vi "prevodni_charakteristika.vi"() -> ()   [LabVIEW 2024]
uses:
  <vilib>/Analysis/baseanly.llb/Mean (DBL).vi
  <instrlib>/EFmeter/EFmeter.lvlib
  <vilib>/Analysis/NI_AALBase.lvlib
panel:
  in  "Dalsi krok\nDalsikrok":bool
  in  "Zpusob rizeni napeti":u16(ring) items=["Sweep", "Manualni", ""]
  in  "VISA EFmeter":refnum<visa-resource-name>
  out "S":dbl
  in  "file path (use dialog)":path
  in  "Prodleva mezi vzorky(ms)":u32
  in  "Prumerovani":bool
  in  "Vzorku na kroků":u16 max=100 step=1
  out "Prevodni charakteristika":cluster{"X":dbl[], "Y":dbl[]}[](graph)
  in  "Clear":bool
  in  "Uložit data":bool
  in  "Start":bool
  in  "VISA  zdroj":refnum<visa-resource-name>
  in  "stop":bool
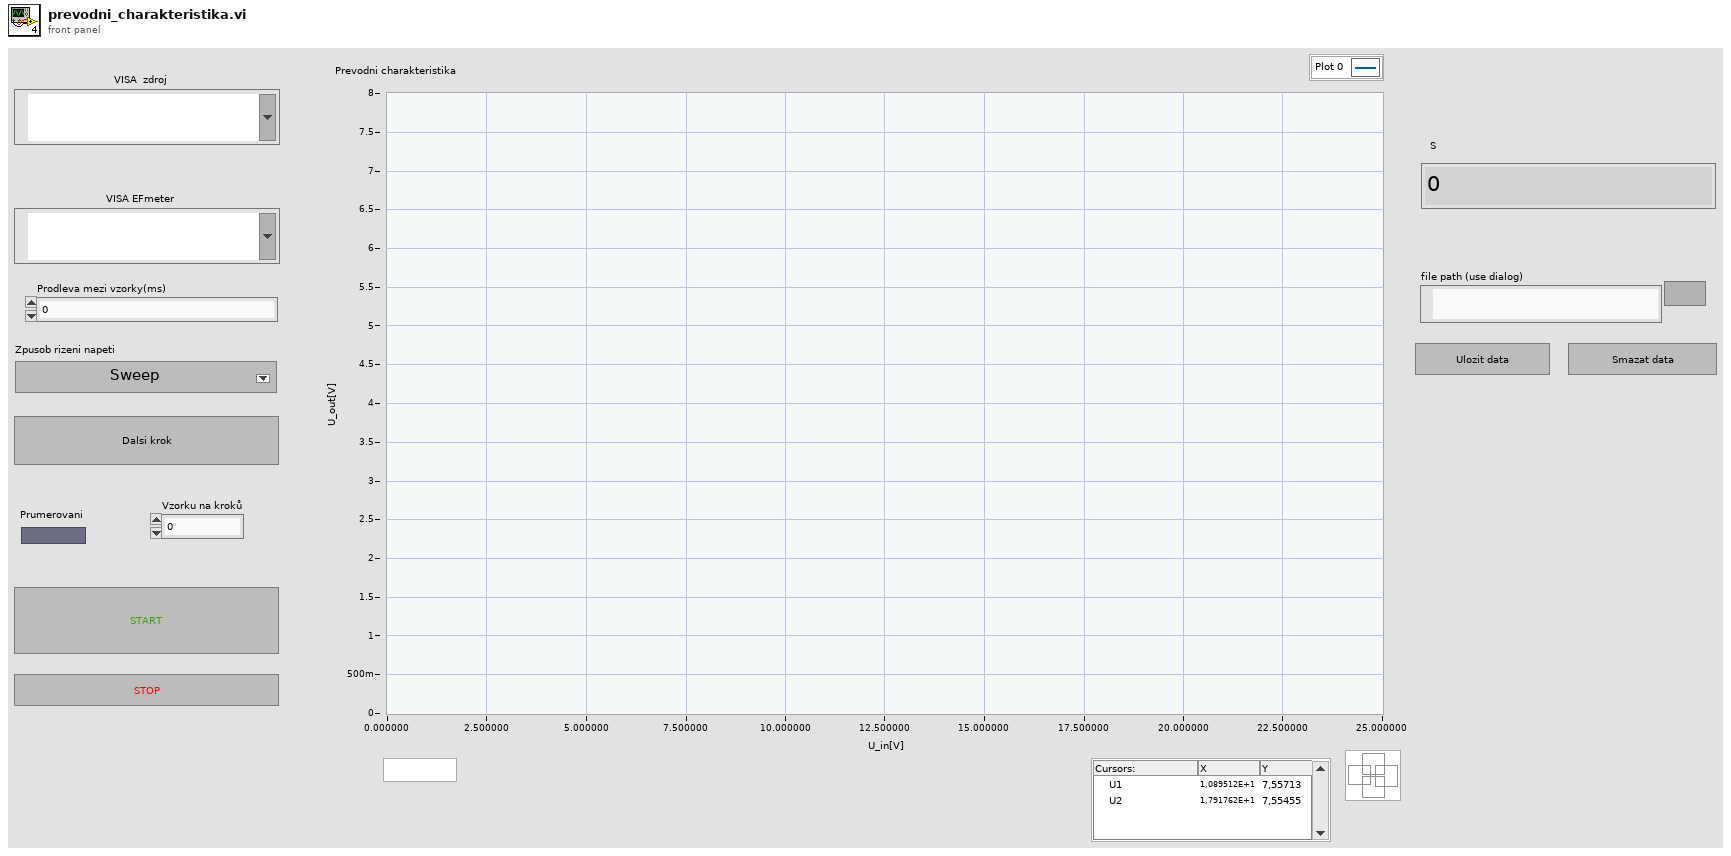
[diagram p1: front panel]
types:
  T1 = enum16{"Default", "Wait", "Refresh", "Measure", "Change input", "Init_meas", "Uloz"}
  T2 = typedef "LVCursorListTypeDef.ctl" = cluster{"Name":string, "Color":u32, "Style":u8, "Point Style":u8, "Name Visible":bool, "Allow Drag":bool, "Cursor Mode":u32, "Plot":i32, "Index":i32, "Position":cluster{"X":dbl, "Y":dbl}, "X Scale":u32, "Y Scale":u32, "Watch Plots":i32[], "Watch All Plots":bool, "Plot Area":i32, "Label Offset":cluster{"X":dbl, "Y":dbl}}[]
  T3 = cluster{"Name":string, "Color":u32, "Style":u8, "Point Style":u8, "Name Visible":bool, "Allow Drag":bool, "Cursor Mode":u32, "Plot":i32, "Index":i32, "Position":cluster{"X":dbl, "Y":dbl}, "X Scale":u32, "Y Scale":u32, "Watch Plots":i32[], "Watch All Plots":bool, "Plot Area":i32, "Label Offset":cluster{"X":dbl, "Y":dbl}}
  T4 = enum16{"open", "replace", "create", "open or create", "replace or create", "replace or create with confirmation"}
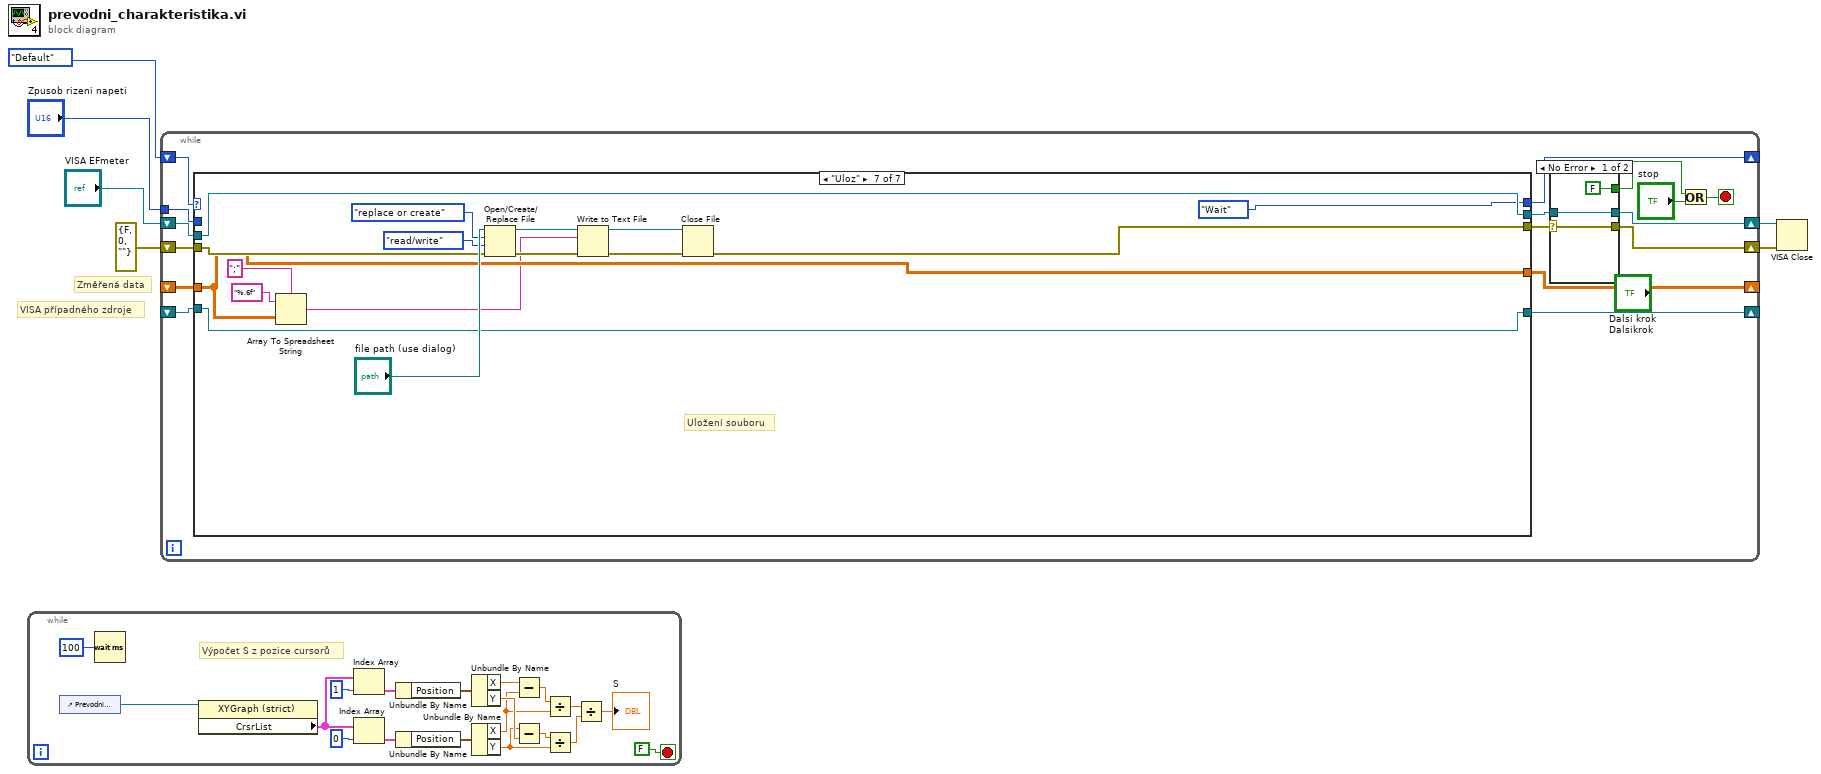
[diagram p0: block diagram]
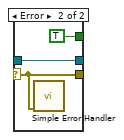
[diagram p2: hidden frame]
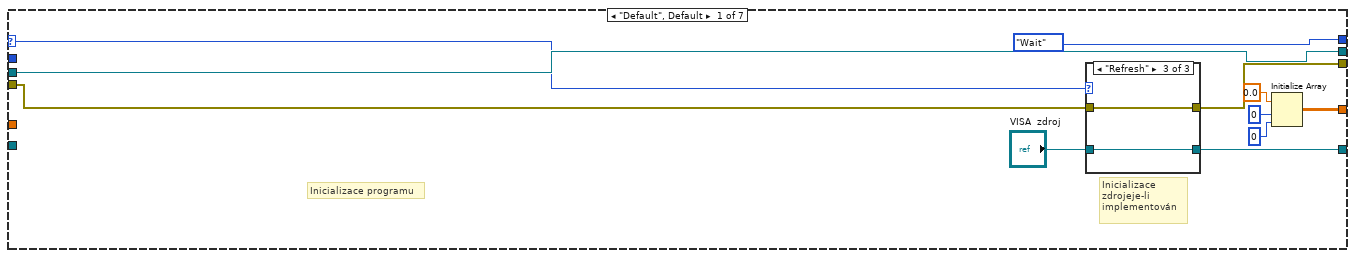
[diagram p3: hidden frame]
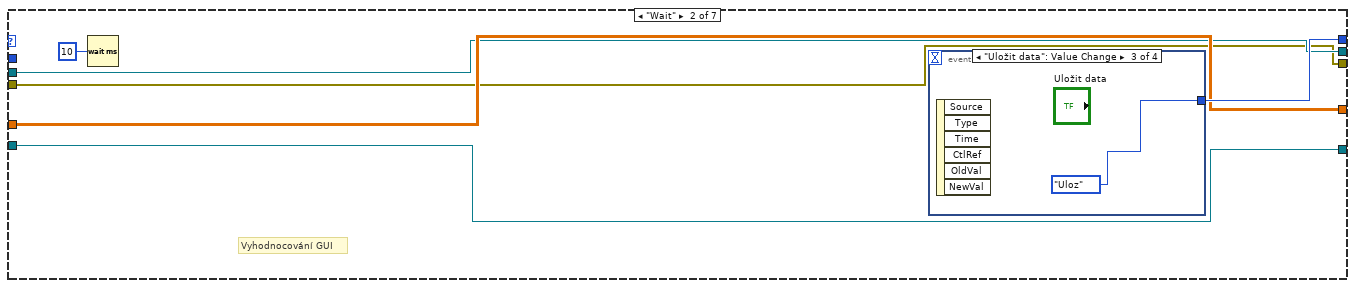
[diagram p6: hidden frame]
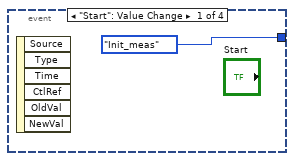
[diagram p7: hidden frame]
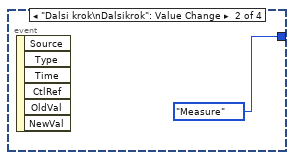
[diagram p8: hidden frame]
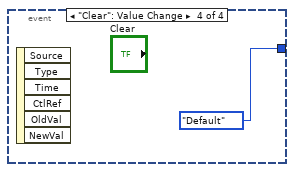
[diagram p9: hidden frame]
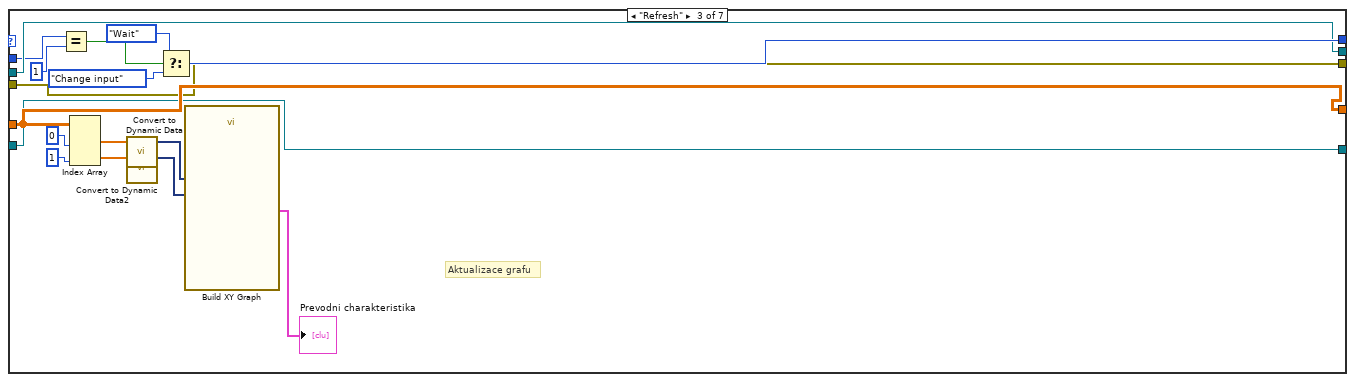
[diagram p10: hidden frame]
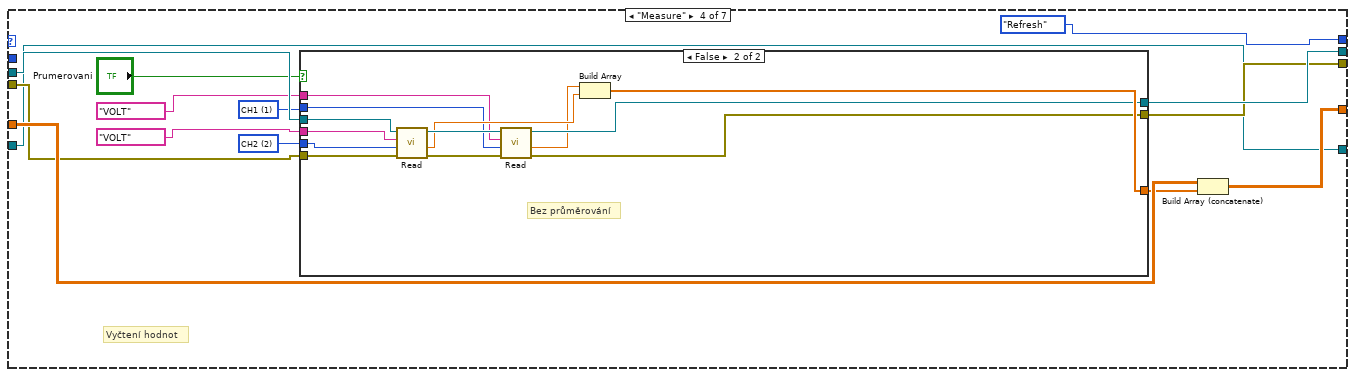
[diagram p11: hidden frame]
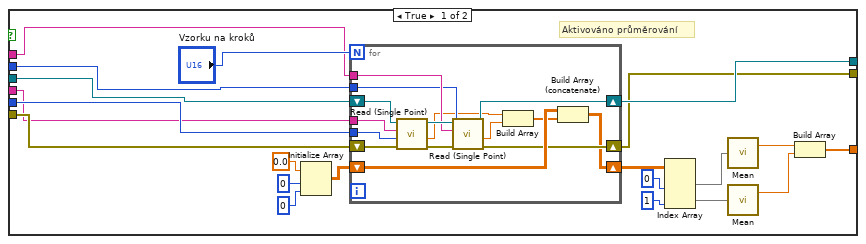
[diagram p12: hidden frame]
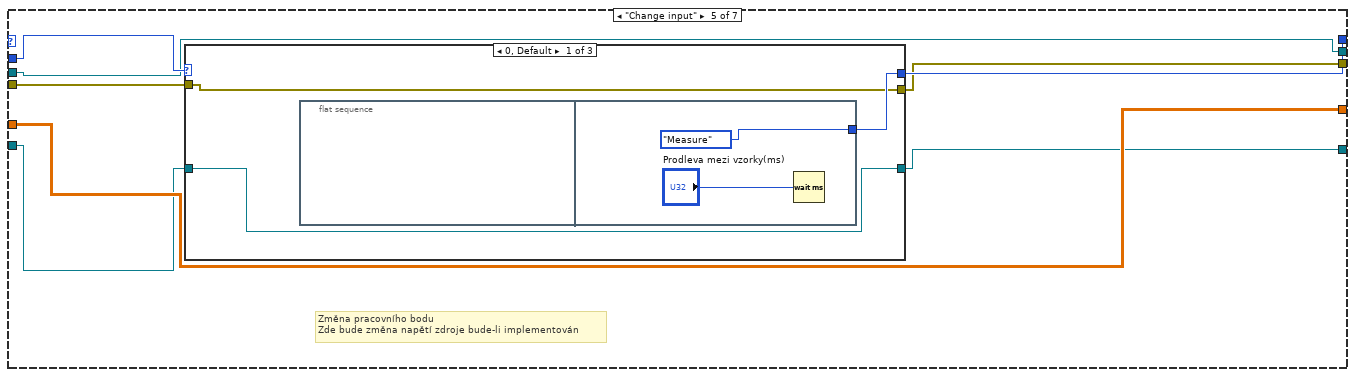
[diagram p13: hidden frame]
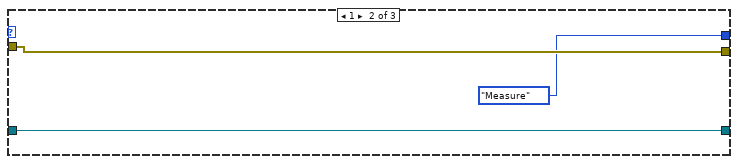
[diagram p14: hidden frame]
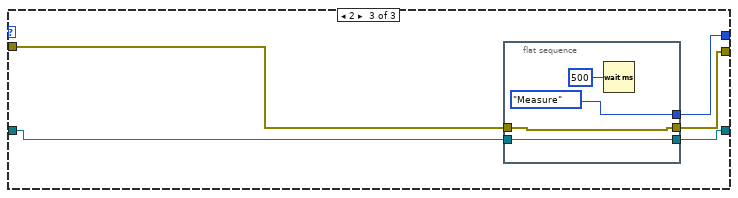
[diagram p15: hidden frame]
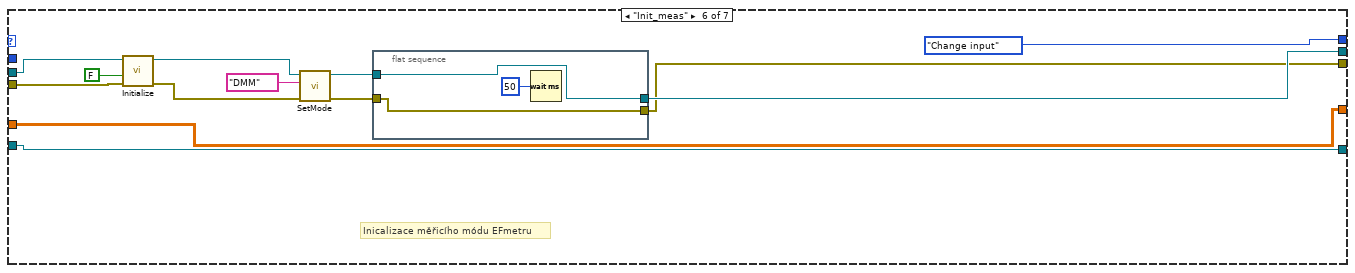
[diagram p16: hidden frame]
diagram:
  # "VISA případného zdroje"
  # "Změřená data"
  n1 = while {
    stop <- FALSE stop-if-true
    # "Výpočet S z pozice cursorů"
    n2 = control-ref of="Prevodni charakteristika"() -> (w23:refnum<vi>)
    n3 = Wait (ms)(milliseconds to wait=u32 100) -> ()  [unwired: 1 out]
    n4 = property class="XYGraph (strict)"(reference=w23) -> ("CrsrList"=w18:T2)  [unwired: 1 in, 2 out]
    n5 = Index Array(array=w18, index=1) -> (element=w20:T3)
    n6 = Index Array(array=w18, index=0) -> (element=w24:T3)
    n7 = Unbundle By Name(w20) -> ("Position"=w21:cluster{"X":dbl, "Y":dbl})
    n8 = Unbundle By Name(w24) -> ("Position"=w25:cluster{"X":dbl, "Y":dbl})
    n9 = Unbundle By Name(w21) -> ("X"=w13:dbl, "Y"=w17:dbl)
    n10 = Unbundle By Name(w25) -> ("X"=w8:dbl, "Y"=w11:dbl)
    n11 = Subtract(x=w13, y=w8) -> (x-y=w9:dbl)
    n12 = Subtract(x=w11, y=w17) -> (x-y=w12:dbl)
    n13 = Divide(x=w9, y=w8) -> (x/y=w7:dbl)
    n14 = Divide(x=w12, y=w11) -> (x/y=w10:dbl)
    n15 = Divide(x=w7, y=w10) -> (x/y=→"S":dbl)
  }
  n16 = while {
    shift-right: [w41] -> _
    shift-left: _ -> [w40]
    shift-right: [w36] -> _
    shift-left: T1."Default" -> [w39]
    shift-right: [w33] -> w4
    shift-left: "VISA EFmeter" -> [w38]
    shift-right: [w26] -> w3
    shift-left: errorcluster {"status"=FALSE, "code"=0, "source"=""} ("error in (no error)") -> [w37]
    tunnel: "Zpusob rizeni napeti" -> [w29]
    shift-right: [w28] -> _
    shift-left: _ -> [w27]
    stop <- w31 stop-if-true
    n17 = case shown="\"Uloz\"" w39 {
      selector: w39 -> [w53 _ _ _ _ _ _]
      tunnel: [w56 w69 w87 w104 w162 w192 w206] -> w41
      tunnel: w40 -> [_ w69 w87 w105 w162 w192 w206]
      tunnel: [T1."Wait" w70 w86 T1."Refresh" w160 T1."Change input" T1."Wait"] -> w36
      tunnel: [w51 w67 w81 w95 w155 w190 w201] -> w35
      tunnel: [w54 w68 w82 w96 w159 w191 w211] -> w34
      tunnel: w38 -> [w54 w68 w82 w102 w159 w188 w211]
      tunnel: w37 -> [w52 w67 w81 w101 w156 w187 w207]
      tunnel: w29 -> [_ _ w79 _ w161 _ _]
      tunnel: [w50 w65 w80 w93 w157 w189 w197] -> w28
      tunnel: w27 -> [_ w65 w80 w93 w158 w189 w197]
      frame "Default", Default {
        # "Inicializace\nzdrojeje-li \nimplementován"
        # "Inicializace programu"
        n18 = case shown="\"Refresh\"" w53 {
          tunnel: w52 -> [w60 w61 w63]
          tunnel: [w60 w61 w63] -> w51
          tunnel: [w59 w62 w64] -> w50
          tunnel: "VISA  zdroj" -> [w59 w62 w64]
          frame "Default", Default {
          }
          frame "Wait" {
          }
          frame "Refresh" {
          }
        }
        n19 = Initialize Array(0.0 ("element"), 0 ("dimension size"), 0 ("dimension size")) -> (w56:dbl[][])
      }
      frame "Wait" {
        # "Vyhodnocování GUI"
        n20 = Wait (ms)(milliseconds to wait=u32 10) -> ()  [unwired: 1 out]
        n21 = event shown="[2] \"Uložit data\": Value Change" {
          selector: _ -> [_ _ _ _]
          dyn-events: _ -> [_ _ _ _]
          timeout: _ -> [_ _ _ _]
          tunnel: [T1."Init_meas" T1."Measure" T1."Uloz" T1."Default"] -> w70
          event "Start": Value Change {
            n22 = event-data() -> ()  [unwired: 1 in, 6 out]
          }
          event "Dalsi krok\nDalsikrok": Value Change {
            n23 = event-data() -> ()  [unwired: 1 in, 6 out]
          }
          event "Uložit data": Value Change {
            n24 = event-data() -> ()  [unwired: 1 in, 6 out]
          }
          event "Clear": Value Change {
            n25 = event-data() -> ()  [unwired: 1 in, 6 out]
          }
        }
      }
      frame "Refresh" {
        # "Aktualizace grafu"
        n26 = Equal?(x=w79, y=u16 1) -> (x = y?=w77:bool)
        n27 = Index Array(array=w87, index (col) #1=0 ("index (row)"), index (col) #2=1 ("index (row)")) -> (element #1=w91:dbl[], element #2=w88:dbl[])  [unwired: 2 in]
        n28 = call "Convert to Dynamic Data"("Array"=w91) -> ("Dynamic Data Type"=w90:dynamicdata)  [unwired: 3 in]
        n29 = call "Convert to Dynamic Data2"("Array"=w88) -> ("Dynamic Data Type"=w89:dynamicdata)  [unwired: 3 in]
        n30 = Select(t=T1."Wait", s=w77, f=T1."Change input") -> (s? t:f=w86:T1)
        n31 = call "Build XY Graph"("Y Input"=w89, "X Input"=w90) -> ("XY Graph"=→"Prevodni charakteristika":cluster{"X":dbl[], "Y":dbl[]}[])  [unwired: 8 in, 1 out]
      }
      frame "Measure" {
        w97 = u16 1 items=["CH2"=2, "CH1"=1] ("Ring")
        w100 = u16 2 items=["CH2"=2, "CH1"=1] ("Ring")
        # "Vyčtení hodnot"
        n32 = case shown="False" "Prumerovani" {
          tunnel: [w108 w154] -> w103
          tunnel: w102 -> [w121 w153]
          tunnel: w101 -> [w120 w150]
          tunnel: w100 -> [w119 w151]
          tunnel: "VOLT" ("Combo Box") -> [w118 w152]
          tunnel: "VOLT" ("Combo Box") -> [w117 w146]
          tunnel: w97 -> [w116 w145]
          tunnel: [w107 w144] -> w96
          tunnel: [w106 w143] -> w95
          frame True {
            # "Aktivováno průměrování"
            n33 = Initialize Array(0.0 ("element"), 0 ("dimension size"), 0 ("dimension size")) -> (w122:dbl[][])
            n34 = for {
              N: "Vzorku na kroků" -> [_]
              shift-right: [w137] -> w107
              shift-left: w121 -> [w138]
              shift-right: [w135] -> w106
              shift-left: w120 -> [w136]
              tunnel: w119 -> [w134]
              tunnel: w118 -> [w133]
              tunnel: w117 -> [w132]
              tunnel: w116 -> [w131]
              shift-right: [w130] -> w115
              shift-left: w122 -> [w139]
              n35 = call <instrlib>:"Read (Single Point).vi"("error in (no error)"=w136, "Ring"=w134, "Combo Box"=w133, "VISA resource name"=w138) -> ("error out"=w140:errorcluster, "Measurement"=w128:dbl, "VISA resource name out"=w141:refnum<visa-resource-name>)  [unwired: 5 in]
              n36 = call <instrlib>:"Read (Single Point).vi"("error in (no error)"=w140, "Ring"=w131, "Combo Box"=w132, "VISA resource name"=w141) -> ("error out"=w135:errorcluster, "Measurement"=w129:dbl, "VISA resource name out"=w137:refnum<visa-resource-name>)  [unwired: 5 in]
              n37 = Build Array(w128, w129) -> (w127:dbl[])
              n38 = Build Array (concatenate)(w139, w127) -> (w130:dbl[][])
            }
            n39 = Index Array(array=w115, index (col) #1=0 ("disabled index (col)"), index (col) #2=1 ("index (col)")) -> (element #1=w114:dbl[], element #2=w113:dbl[])  [unwired: 2 in]
            n40 = call-poly <vilib>:"Mean.vi"("X"=w114) -> ("mean"=w110:dbl)  [unwired: 1 out]
            n41 = call-poly <vilib>:"Mean.vi"("X"=w113) -> ("mean"=w109:dbl)  [unwired: 1 out]
            n42 = Build Array(w110, w109) -> (w108:dbl[])
          }
          frame False {
            # "Bez průměrování"
            n43 = call-poly <instrlib>:"Read.vi"("error in (no error)"=w150, "Ring"=w151, "Combo Box"=w152, "VISA resource name"=w153) -> ("error out"=w148:errorcluster, "Measurement"=w147:dbl, "VISA resource name out"=w149:refnum<visa-resource-name>)  [unwired: 5 in]
            n44 = call-poly <instrlib>:"Read.vi"("error in (no error)"=w148, "Ring"=w145, "Combo Box"=w146, "VISA resource name"=w149) -> ("error out"=w143:errorcluster, "Measurement"=w142:dbl, "VISA resource name out"=w144:refnum<visa-resource-name>)  [unwired: 5 in]
            n45 = Build Array(w142, w147) -> (w154:dbl[])
          }
        }
        n46 = Build Array (concatenate)(w105, w103) -> (w104:dbl[][])
      }
      frame "Change input" {
        # "Změna pracovního bodu\nZde bude změna napětí zdroje bude-li implementován"
        n47 = case shown="0, Default" w161 {
          tunnel: [w165 T1."Measure" w173] -> w160
          tunnel: w158 -> [w164 w170 w172]
          tunnel: [w164 w170 w174] -> w157
          tunnel: w156 -> [w163 w169 w171]
          tunnel: [w163 w169 w175] -> w155
          frame 0, Default {
            n48 = flat-sequence {
              tunnel: [T1."Measure"] -> w165
              frame #0 {
              }
              frame #1 {
                n49 = Wait (ms)(milliseconds to wait="Prodleva mezi vzorky(ms)") -> ()  [unwired: 1 out]
              }
            }
          }
          frame 1 {
          }
          frame 2 {
            n50 = flat-sequence {
              tunnel: w171 -> [w179]
              tunnel: [w179] -> w175
              tunnel: [w178] -> w174
              tunnel: w172 -> [w178]
              tunnel: [T1."Measure"] -> w173
              frame #0 {
                n51 = Wait (ms)(milliseconds to wait=u32 500) -> ()  [unwired: 1 out]
              }
            }
          }
        }
      }
      frame "Init_meas" {
        # "Inicalizace měřicího módu EFmetru"
        n52 = call <instrlib>:"Initialize.vi"("error in (no error)"=w187, "Reset (True)"=FALSE, "VISA resource name"=w188) -> ("error out"=w184:errorcluster, "VISA resource name out"=w185:refnum<visa-resource-name>)  [unwired: 7 in]
        n53 = call <instrlib>:"SetMode.vi"("error in (no error)"=w184, "Combo Box"="DMM", "VISA resource name"=w185) -> ("error out"=w183:errorcluster, "VISA resource name out"=w182:refnum<visa-resource-name>)  [unwired: 7 in]
        n54 = flat-sequence {
          tunnel: [w194] -> w191
          tunnel: w182 -> [w194]
          tunnel: w183 -> [w193]
          tunnel: [w193] -> w190
          frame #0 {
            n55 = Wait (ms)(milliseconds to wait=u32 50) -> ()  [unwired: 1 out]
          }
        }
      }
      frame "Uloz" {
        # "Uložení souboru"
        n56 = Array To Spreadsheet String(delimiter (Tab)=";", array=w206, 3:"%.6f" ("format string")) -> (spreadsheet string=w198:string)
        n57 = Open/Create/Replace File(file path (use dialog)="file path (use dialog)", error in=w207, operation (0:open)=T4."replace or create", access (0:read/write)=enum16{"read/write", "read-only", "write-only"}."read/write") -> (refnum out=w200:refnum<file>, error out=w203:errorcluster)  [unwired: 2 in, 1 out]
        n58 = Write to Text File(file (use dialog)=w200, text=w198, error in=w203) -> (refnum out=w199:refnum<file>, error out=w202:errorcluster)  [unwired: 1 in, 1 out]
        n59 = Close File(refnum=w199, error in=w202) -> (error out=w201:errorcluster)  [unwired: 1 out]
      }
    }
    n60 = case shown="No Error" w35 {
      selector: w35 -> [w42 w45]
      tunnel: w34 -> [w44 w47]
      tunnel: [w44 w47] -> w33
      tunnel: [w42 w45] -> w26
      tunnel: [FALSE TRUE] -> w30
      frame No Error {
      }
      frame Error {
        n61 = call <vilib>:"Simple Error Handler.vi"("error in (no error)"=w45) -> ()  [unwired: 4 in, 5 out]
      }
    }
    n62 = Or(x=w30, y="stop") -> (x .or. y?=w31:bool)
  }
  n63 = VISA Close(VISA resource name=w4, error in (no error)=w3) -> ()  [unwired: 1 out]
